vi "subChannelFreq.vi"(1 "Channel":i32=3) -> (0 "Freq.":dbl)   [LabVIEW 2014]
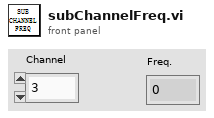
[diagram p1: front panel]
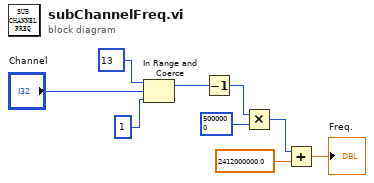
[diagram p0: block diagram]
diagram:
  n1 = In Range and Coerce(upper limit=13 ("lower limit"), x="Channel", lower limit=1) -> (coerced(x)=w6:i32)  [unwired: 1 out]
  n2 = Decrement(x=w6) -> (x-1=w5:i32)
  n3 = Multiply(x=w5, y=5000000) -> (x*y=w3:i32)
  n4 = Add(x=w3, y=2412000000.0) -> (x+y=→"Freq.":dbl)
